vi "Configure.vi"(8 "error in (no error)":errorcluster, 11 "Data Rate [S/s]":u32) -> (0 "error out":errorcluster)   [LabVIEW 2017, in "MCSA_9065_API.lvlib"]
uses:
  <vilib>/addons/InsightCM/Devices/Shared/Mcsa/Fpga/McsaAcquire/subVIs/McsaAPI_9065/MCSA_9065_API.lvlib
  <vilib>/eio/EIOPropertyNode/EIOPropertyNode.xnode
  <vilib>/rvi/eio/common/nirviEmuTemplatePropertyGet_errors.vi
  <vilib>/rvi/eio/common/nirviEmuTemplatePropertyGet_noerrors.vi
  <vilib>/rvi/eio/common/nirviEmuTemplatePropertySet_errors.vi
  <vilib>/rvi/eio/common/nirviEmuTemplatePropertySet_noerrors.vi
  <vilib>/LabVIEW Targets/FPGA/cRIO/shared/nicrio_ModuleControls/nicrio_cRIO-9239_DataRatesRing.ctl
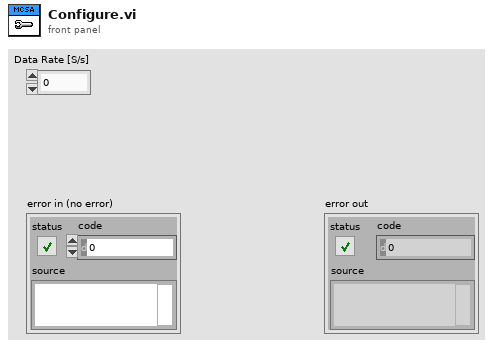
[diagram p1: front panel]
types:
  T1 = typedef "nicrio_cRIO-9239_DataRatesRing.ctl" = u8
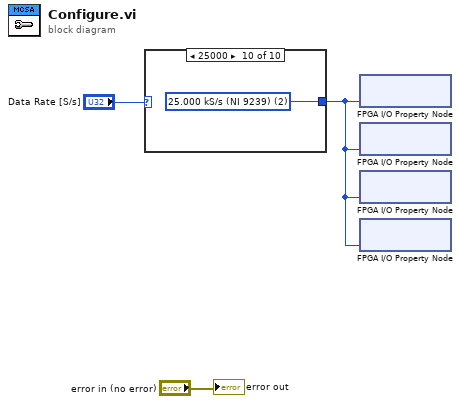
[diagram p0: block diagram]
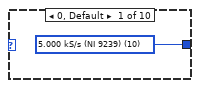
[diagram p2: hidden frame]
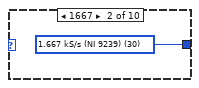
[diagram p3: hidden frame]
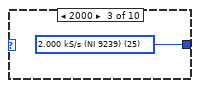
[diagram p4: hidden frame]
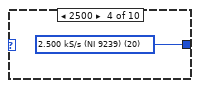
[diagram p5: hidden frame]
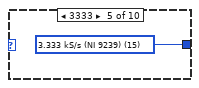
[diagram p6: hidden frame]
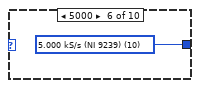
[diagram p7: hidden frame]
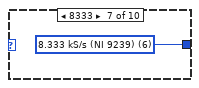
[diagram p8: hidden frame]
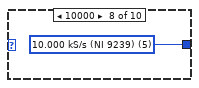
[diagram p9: hidden frame]
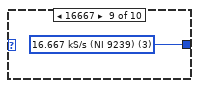
[diagram p10: hidden frame]
diagram:
  n1 = case shown="25000" "Data Rate [S/s]" {
    tunnel: [w4 w5 w6 w7 w8 w9 w10 w11 w12 w13] -> w1
    frame 0, Default {
      w4 = T1 10 items=["50.000 kS/s (NI 9239)"=1, "25.000 kS/s (NI 9239)"=2, "16.667 kS/s (NI 9239)"=3, "12.500 kS/s (NI 9239)"=4, "10.000 kS/s (NI 9239)"=5, "8.333 kS/s (NI 9239)"=6, "7.143 kS/s (NI 9239)"=7, "6.250 kS/s (NI 9239)"=8, "5.556 kS/s (NI 9239)"=9, "5.000 kS/s (NI 9239)"=10, "4.545 kS/s (NI 9239)"=11, "4.167 kS/s (NI 9239)"=12, "3.846 kS/s (NI 9239)"=13, "3.571 kS/s (NI 9239)"=14, "3.333 kS/s (NI 9239)"=15, "3.125 kS/s (NI 9239)"=16, "2.941 kS/s (NI 9239)"=17, "2.778 kS/s (NI 9239)"=18, "2.632 kS/s (NI 9239)"=19, "2.500 kS/s (NI 9239)"=20, "2.381 kS/s (NI 9239)"=21, "2.273 kS/s (NI 9239)"=22, "2.174 kS/s (NI 9239)"=23, "2.083 kS/s (NI 9239)"=24, "2.000 kS/s (NI 9239)"=25, "1.923 kS/s (NI 9239)"=26, "1.852 kS/s (NI 9239)"=27, "1.786 kS/s (NI 9239)"=28, "1.724 kS/s (NI 9239)"=29, "1.667 kS/s (NI 9239)"=30, "1.613 kS/s (NI 9239)"=31] ("Data Rate")
    }
    frame 1667 {
      w5 = T1 30 items=["50.000 kS/s (NI 9239)"=1, "25.000 kS/s (NI 9239)"=2, "16.667 kS/s (NI 9239)"=3, "12.500 kS/s (NI 9239)"=4, "10.000 kS/s (NI 9239)"=5, "8.333 kS/s (NI 9239)"=6, "7.143 kS/s (NI 9239)"=7, "6.250 kS/s (NI 9239)"=8, "5.556 kS/s (NI 9239)"=9, "5.000 kS/s (NI 9239)"=10, "4.545 kS/s (NI 9239)"=11, "4.167 kS/s (NI 9239)"=12, "3.846 kS/s (NI 9239)"=13, "3.571 kS/s (NI 9239)"=14, "3.333 kS/s (NI 9239)"=15, "3.125 kS/s (NI 9239)"=16, "2.941 kS/s (NI 9239)"=17, "2.778 kS/s (NI 9239)"=18, "2.632 kS/s (NI 9239)"=19, "2.500 kS/s (NI 9239)"=20, "2.381 kS/s (NI 9239)"=21, "2.273 kS/s (NI 9239)"=22, "2.174 kS/s (NI 9239)"=23, "2.083 kS/s (NI 9239)"=24, "2.000 kS/s (NI 9239)"=25, "1.923 kS/s (NI 9239)"=26, "1.852 kS/s (NI 9239)"=27, "1.786 kS/s (NI 9239)"=28, "1.724 kS/s (NI 9239)"=29, "1.667 kS/s (NI 9239)"=30, "1.613 kS/s (NI 9239)"=31] ("Data Rate")
    }
    frame 2000 {
      w6 = T1 25 items=["50.000 kS/s (NI 9239)"=1, "25.000 kS/s (NI 9239)"=2, "16.667 kS/s (NI 9239)"=3, "12.500 kS/s (NI 9239)"=4, "10.000 kS/s (NI 9239)"=5, "8.333 kS/s (NI 9239)"=6, "7.143 kS/s (NI 9239)"=7, "6.250 kS/s (NI 9239)"=8, "5.556 kS/s (NI 9239)"=9, "5.000 kS/s (NI 9239)"=10, "4.545 kS/s (NI 9239)"=11, "4.167 kS/s (NI 9239)"=12, "3.846 kS/s (NI 9239)"=13, "3.571 kS/s (NI 9239)"=14, "3.333 kS/s (NI 9239)"=15, "3.125 kS/s (NI 9239)"=16, "2.941 kS/s (NI 9239)"=17, "2.778 kS/s (NI 9239)"=18, "2.632 kS/s (NI 9239)"=19, "2.500 kS/s (NI 9239)"=20, "2.381 kS/s (NI 9239)"=21, "2.273 kS/s (NI 9239)"=22, "2.174 kS/s (NI 9239)"=23, "2.083 kS/s (NI 9239)"=24, "2.000 kS/s (NI 9239)"=25, "1.923 kS/s (NI 9239)"=26, "1.852 kS/s (NI 9239)"=27, "1.786 kS/s (NI 9239)"=28, "1.724 kS/s (NI 9239)"=29, "1.667 kS/s (NI 9239)"=30, "1.613 kS/s (NI 9239)"=31] ("Data Rate")
    }
    frame 2500 {
      w7 = T1 20 items=["50.000 kS/s (NI 9239)"=1, "25.000 kS/s (NI 9239)"=2, "16.667 kS/s (NI 9239)"=3, "12.500 kS/s (NI 9239)"=4, "10.000 kS/s (NI 9239)"=5, "8.333 kS/s (NI 9239)"=6, "7.143 kS/s (NI 9239)"=7, "6.250 kS/s (NI 9239)"=8, "5.556 kS/s (NI 9239)"=9, "5.000 kS/s (NI 9239)"=10, "4.545 kS/s (NI 9239)"=11, "4.167 kS/s (NI 9239)"=12, "3.846 kS/s (NI 9239)"=13, "3.571 kS/s (NI 9239)"=14, "3.333 kS/s (NI 9239)"=15, "3.125 kS/s (NI 9239)"=16, "2.941 kS/s (NI 9239)"=17, "2.778 kS/s (NI 9239)"=18, "2.632 kS/s (NI 9239)"=19, "2.500 kS/s (NI 9239)"=20, "2.381 kS/s (NI 9239)"=21, "2.273 kS/s (NI 9239)"=22, "2.174 kS/s (NI 9239)"=23, "2.083 kS/s (NI 9239)"=24, "2.000 kS/s (NI 9239)"=25, "1.923 kS/s (NI 9239)"=26, "1.852 kS/s (NI 9239)"=27, "1.786 kS/s (NI 9239)"=28, "1.724 kS/s (NI 9239)"=29, "1.667 kS/s (NI 9239)"=30, "1.613 kS/s (NI 9239)"=31] ("Data Rate")
    }
    frame 3333 {
      w8 = T1 15 items=["50.000 kS/s (NI 9239)"=1, "25.000 kS/s (NI 9239)"=2, "16.667 kS/s (NI 9239)"=3, "12.500 kS/s (NI 9239)"=4, "10.000 kS/s (NI 9239)"=5, "8.333 kS/s (NI 9239)"=6, "7.143 kS/s (NI 9239)"=7, "6.250 kS/s (NI 9239)"=8, "5.556 kS/s (NI 9239)"=9, "5.000 kS/s (NI 9239)"=10, "4.545 kS/s (NI 9239)"=11, "4.167 kS/s (NI 9239)"=12, "3.846 kS/s (NI 9239)"=13, "3.571 kS/s (NI 9239)"=14, "3.333 kS/s (NI 9239)"=15, "3.125 kS/s (NI 9239)"=16, "2.941 kS/s (NI 9239)"=17, "2.778 kS/s (NI 9239)"=18, "2.632 kS/s (NI 9239)"=19, "2.500 kS/s (NI 9239)"=20, "2.381 kS/s (NI 9239)"=21, "2.273 kS/s (NI 9239)"=22, "2.174 kS/s (NI 9239)"=23, "2.083 kS/s (NI 9239)"=24, "2.000 kS/s (NI 9239)"=25, "1.923 kS/s (NI 9239)"=26, "1.852 kS/s (NI 9239)"=27, "1.786 kS/s (NI 9239)"=28, "1.724 kS/s (NI 9239)"=29, "1.667 kS/s (NI 9239)"=30, "1.613 kS/s (NI 9239)"=31] ("Data Rate")
    }
    frame 5000 {
      w9 = T1 10 items=["50.000 kS/s (NI 9239)"=1, "25.000 kS/s (NI 9239)"=2, "16.667 kS/s (NI 9239)"=3, "12.500 kS/s (NI 9239)"=4, "10.000 kS/s (NI 9239)"=5, "8.333 kS/s (NI 9239)"=6, "7.143 kS/s (NI 9239)"=7, "6.250 kS/s (NI 9239)"=8, "5.556 kS/s (NI 9239)"=9, "5.000 kS/s (NI 9239)"=10, "4.545 kS/s (NI 9239)"=11, "4.167 kS/s (NI 9239)"=12, "3.846 kS/s (NI 9239)"=13, "3.571 kS/s (NI 9239)"=14, "3.333 kS/s (NI 9239)"=15, "3.125 kS/s (NI 9239)"=16, "2.941 kS/s (NI 9239)"=17, "2.778 kS/s (NI 9239)"=18, "2.632 kS/s (NI 9239)"=19, "2.500 kS/s (NI 9239)"=20, "2.381 kS/s (NI 9239)"=21, "2.273 kS/s (NI 9239)"=22, "2.174 kS/s (NI 9239)"=23, "2.083 kS/s (NI 9239)"=24, "2.000 kS/s (NI 9239)"=25, "1.923 kS/s (NI 9239)"=26, "1.852 kS/s (NI 9239)"=27, "1.786 kS/s (NI 9239)"=28, "1.724 kS/s (NI 9239)"=29, "1.667 kS/s (NI 9239)"=30, "1.613 kS/s (NI 9239)"=31] ("Data Rate")
    }
    frame 8333 {
      w10 = T1 6 items=["50.000 kS/s (NI 9239)"=1, "25.000 kS/s (NI 9239)"=2, "16.667 kS/s (NI 9239)"=3, "12.500 kS/s (NI 9239)"=4, "10.000 kS/s (NI 9239)"=5, "8.333 kS/s (NI 9239)"=6, "7.143 kS/s (NI 9239)"=7, "6.250 kS/s (NI 9239)"=8, "5.556 kS/s (NI 9239)"=9, "5.000 kS/s (NI 9239)"=10, "4.545 kS/s (NI 9239)"=11, "4.167 kS/s (NI 9239)"=12, "3.846 kS/s (NI 9239)"=13, "3.571 kS/s (NI 9239)"=14, "3.333 kS/s (NI 9239)"=15, "3.125 kS/s (NI 9239)"=16, "2.941 kS/s (NI 9239)"=17, "2.778 kS/s (NI 9239)"=18, "2.632 kS/s (NI 9239)"=19, "2.500 kS/s (NI 9239)"=20, "2.381 kS/s (NI 9239)"=21, "2.273 kS/s (NI 9239)"=22, "2.174 kS/s (NI 9239)"=23, "2.083 kS/s (NI 9239)"=24, "2.000 kS/s (NI 9239)"=25, "1.923 kS/s (NI 9239)"=26, "1.852 kS/s (NI 9239)"=27, "1.786 kS/s (NI 9239)"=28, "1.724 kS/s (NI 9239)"=29, "1.667 kS/s (NI 9239)"=30, "1.613 kS/s (NI 9239)"=31] ("Data Rate")
    }
    frame 10000 {
      w11 = T1 5 items=["50.000 kS/s (NI 9239)"=1, "25.000 kS/s (NI 9239)"=2, "16.667 kS/s (NI 9239)"=3, "12.500 kS/s (NI 9239)"=4, "10.000 kS/s (NI 9239)"=5, "8.333 kS/s (NI 9239)"=6, "7.143 kS/s (NI 9239)"=7, "6.250 kS/s (NI 9239)"=8, "5.556 kS/s (NI 9239)"=9, "5.000 kS/s (NI 9239)"=10, "4.545 kS/s (NI 9239)"=11, "4.167 kS/s (NI 9239)"=12, "3.846 kS/s (NI 9239)"=13, "3.571 kS/s (NI 9239)"=14, "3.333 kS/s (NI 9239)"=15, "3.125 kS/s (NI 9239)"=16, "2.941 kS/s (NI 9239)"=17, "2.778 kS/s (NI 9239)"=18, "2.632 kS/s (NI 9239)"=19, "2.500 kS/s (NI 9239)"=20, "2.381 kS/s (NI 9239)"=21, "2.273 kS/s (NI 9239)"=22, "2.174 kS/s (NI 9239)"=23, "2.083 kS/s (NI 9239)"=24, "2.000 kS/s (NI 9239)"=25, "1.923 kS/s (NI 9239)"=26, "1.852 kS/s (NI 9239)"=27, "1.786 kS/s (NI 9239)"=28, "1.724 kS/s (NI 9239)"=29, "1.667 kS/s (NI 9239)"=30, "1.613 kS/s (NI 9239)"=31] ("Data Rate")
    }
    frame 16667 {
      w12 = T1 3 items=["50.000 kS/s (NI 9239)"=1, "25.000 kS/s (NI 9239)"=2, "16.667 kS/s (NI 9239)"=3, "12.500 kS/s (NI 9239)"=4, "10.000 kS/s (NI 9239)"=5, "8.333 kS/s (NI 9239)"=6, "7.143 kS/s (NI 9239)"=7, "6.250 kS/s (NI 9239)"=8, "5.556 kS/s (NI 9239)"=9, "5.000 kS/s (NI 9239)"=10, "4.545 kS/s (NI 9239)"=11, "4.167 kS/s (NI 9239)"=12, "3.846 kS/s (NI 9239)"=13, "3.571 kS/s (NI 9239)"=14, "3.333 kS/s (NI 9239)"=15, "3.125 kS/s (NI 9239)"=16, "2.941 kS/s (NI 9239)"=17, "2.778 kS/s (NI 9239)"=18, "2.632 kS/s (NI 9239)"=19, "2.500 kS/s (NI 9239)"=20, "2.381 kS/s (NI 9239)"=21, "2.273 kS/s (NI 9239)"=22, "2.174 kS/s (NI 9239)"=23, "2.083 kS/s (NI 9239)"=24, "2.000 kS/s (NI 9239)"=25, "1.923 kS/s (NI 9239)"=26, "1.852 kS/s (NI 9239)"=27, "1.786 kS/s (NI 9239)"=28, "1.724 kS/s (NI 9239)"=29, "1.667 kS/s (NI 9239)"=30, "1.613 kS/s (NI 9239)"=31] ("Data Rate")
    }
    frame 25000 {
      w13 = T1 2 items=["50.000 kS/s (NI 9239)"=1, "25.000 kS/s (NI 9239)"=2, "16.667 kS/s (NI 9239)"=3, "12.500 kS/s (NI 9239)"=4, "10.000 kS/s (NI 9239)"=5, "8.333 kS/s (NI 9239)"=6, "7.143 kS/s (NI 9239)"=7, "6.250 kS/s (NI 9239)"=8, "5.556 kS/s (NI 9239)"=9, "5.000 kS/s (NI 9239)"=10, "4.545 kS/s (NI 9239)"=11, "4.167 kS/s (NI 9239)"=12, "3.846 kS/s (NI 9239)"=13, "3.571 kS/s (NI 9239)"=14, "3.333 kS/s (NI 9239)"=15, "3.125 kS/s (NI 9239)"=16, "2.941 kS/s (NI 9239)"=17, "2.778 kS/s (NI 9239)"=18, "2.632 kS/s (NI 9239)"=19, "2.500 kS/s (NI 9239)"=20, "2.381 kS/s (NI 9239)"=21, "2.273 kS/s (NI 9239)"=22, "2.174 kS/s (NI 9239)"=23, "2.083 kS/s (NI 9239)"=24, "2.000 kS/s (NI 9239)"=25, "1.923 kS/s (NI 9239)"=26, "1.852 kS/s (NI 9239)"=27, "1.786 kS/s (NI 9239)"=28, "1.724 kS/s (NI 9239)"=29, "1.667 kS/s (NI 9239)"=30, "1.613 kS/s (NI 9239)"=31] ("Data Rate")
    }
  }
  n2 = xnode "FPGA I/O Property Node"("Data Rate"=w1) -> ()  [unwired: 2 in, 2 out]
  n3 = xnode "FPGA I/O Property Node"("Data Rate"=w1) -> ()  [unwired: 2 in, 2 out]
  n4 = xnode "FPGA I/O Property Node"("Data Rate"=w1) -> ()  [unwired: 2 in, 2 out]
  n5 = xnode "FPGA I/O Property Node"("Data Rate"=w1) -> ()  [unwired: 2 in, 2 out]
  "error out" <- "error in (no error)"
